vi "Log Data.vi"(0 "Log Data":bool[](array[boolean]), 1 "Log AKLH":bool[](array[boolean]), 2 "Data Log Dirs":path[](array[path]), 3 "AKLH Today Dirs":path[](array[path]), 4 "Record Time (sec)":dbl, 5 "Target Speed":u16, 6 "Test Profile":T4[](array[typedef]) {"Pump Cmds"."Pump 6\nCmd" min=0 format="%#.1f"; "Pump Cmds"."Pump 5\nCmd" min=0 format="%#.1f"; "Pump Cmds"."Pump 4\nCmd" min=0 format="%#.1f"; "Pump Cmds"."Pump 3\nCmd" min=0 format="%#.1f"; "Pump Cmds"."Pump 2\nCmd" min=0 format="%#.1f"; "Pump Cmds"."Pump 1\nCmd" min=0 format="%#.1f"; "Temp\nCmd" min=-60 max=100; "Pressure\nCmd" max=20; "PS\nCmd" min=0 max=20 format="%#.2f"; "Time (s)" min=0.0 step=0.01 format="%#.2g"}, 7 "Current Step":i32=2, 8 "Pump Data":T3={"Voltages"=[0.015201568603515625, 0.00335693359375, 0.003021240234375, 0.12260055541992188, 0.06085968017578125, 0.052234649658203125], "PumpCurrent"=[0.015201568603515625, 0.00335693359375, 0.003021240234375, 0.12260055541992188, 0.06085968017578125, 0.052234649658203125], "Speed"=[0.0, 0.0, 0.0, 0.0, 0.0, 0.0], "ControllerCurrent"=[0.015201568603515625, 0.00335693359375, 0.003021240234375, 0.12260055541992188, 0.06085968017578125, 0.052234649658203125], "Pressure"=[0.015201568603515625, 0.00335693359375, 0.003021240234375, 0.12260055541992188, 0.06085968017578125, 0.052234649658203125], "Flow"=[0.0, 0.0, 0.0, 0.125, 0.0625, 0.0625], "Elapsed Time (Display)"=[7.1, 7.1, 7.1, 458133.45, 458138.85000000003, 458126.75], "Avg Pressure"=0.0, "Avg Speed"=0.0, "Elapsed Time"=[4074.9003000000002, 4074.9003000000002, 4074.9003000000002, 4074.9003000000002, 4074.9003000000002, 4074.9003000000002], "Diagnostic"=[0.0, 0.0, 0.0, 0.0, 0.0, 0.0]} {"Diagnostic" format="%#.0f"; "Elapsed Time" format="%<%H:%M:%S>t"; "Elapsed Time (Display)" format="%<%H:%M:%S>t"; "Speed" format="%#_4f"; "ControllerCurrent" format="%#.1g"; "Pressure" format="%#.0f"; "Flow" format="%#.0f"; "PumpCurrent" format="%#.1g"; "Voltages" format="%#.0f"}, 9 "Tank CMDs":T1, 10 "Tank Data":T2 {"PS Actual (V):" format="%.2f"; "Temp1" format="%#_2g"; "Temp2" format="%#_2g"}, 11 "AKLH Filename":string, 13 "3 Pump Tank":bool) -> ()   [LabVIEW 2019]
uses:
  Type Defs/Test Step.ctl
  Type Defs/Pump Cmds.ctl
  Controls/Pump Data.ctl
  Controls/Tank Data.ctl
  Controls/Tank CMDs.ctl
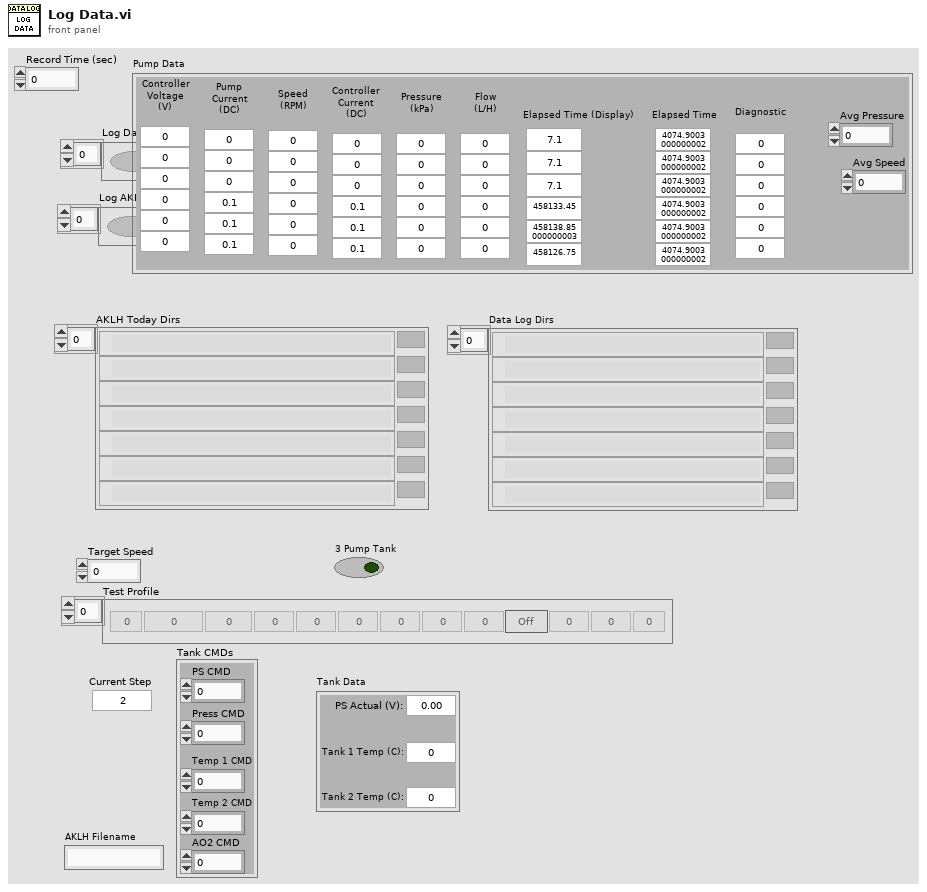
[diagram p1: front panel]
types:
  T1 = typedef "Tank CMDs.ctl" = cluster{"PS CMD":dbl, "Press CMD":dbl, "Temp 1 CMD":dbl, "Temp 2 CMD":dbl, "AO2 CMD":dbl}
  T2 = typedef "Tank Data.ctl" = cluster{"PS Actual (V):":dbl, "Temp1":dbl, "Temp2":dbl}
  T3 = typedef "Pump Data.ctl" = cluster{"Voltages":dbl[], "PumpCurrent":dbl[], "Speed":dbl[], "ControllerCurrent":dbl[], "Pressure":dbl[], "Flow":dbl[], "Elapsed Time (Display)":dbl[], "Avg Pressure":dbl, "Avg Speed":dbl, "Elapsed Time":dbl[], "Diagnostic":dbl[]}
  T4 = typedef "Test Step.ctl" = cluster{"Step":u8, "Time (s)":dbl, "Target\nSpeed":u16, "Pump Cmds":T5, "Relays":bool, "PS\nCmd":sgl, "Pressure\nCmd":u16, "Temp\nCmd":i16}
  T5 = typedef "Pump Cmds.ctl" = cluster{"Pump 1\nCmd":sgl, "Pump 2\nCmd":sgl, "Pump 3\nCmd":sgl, "Pump 4\nCmd":sgl, "Pump 5\nCmd":sgl, "Pump 6\nCmd":sgl}
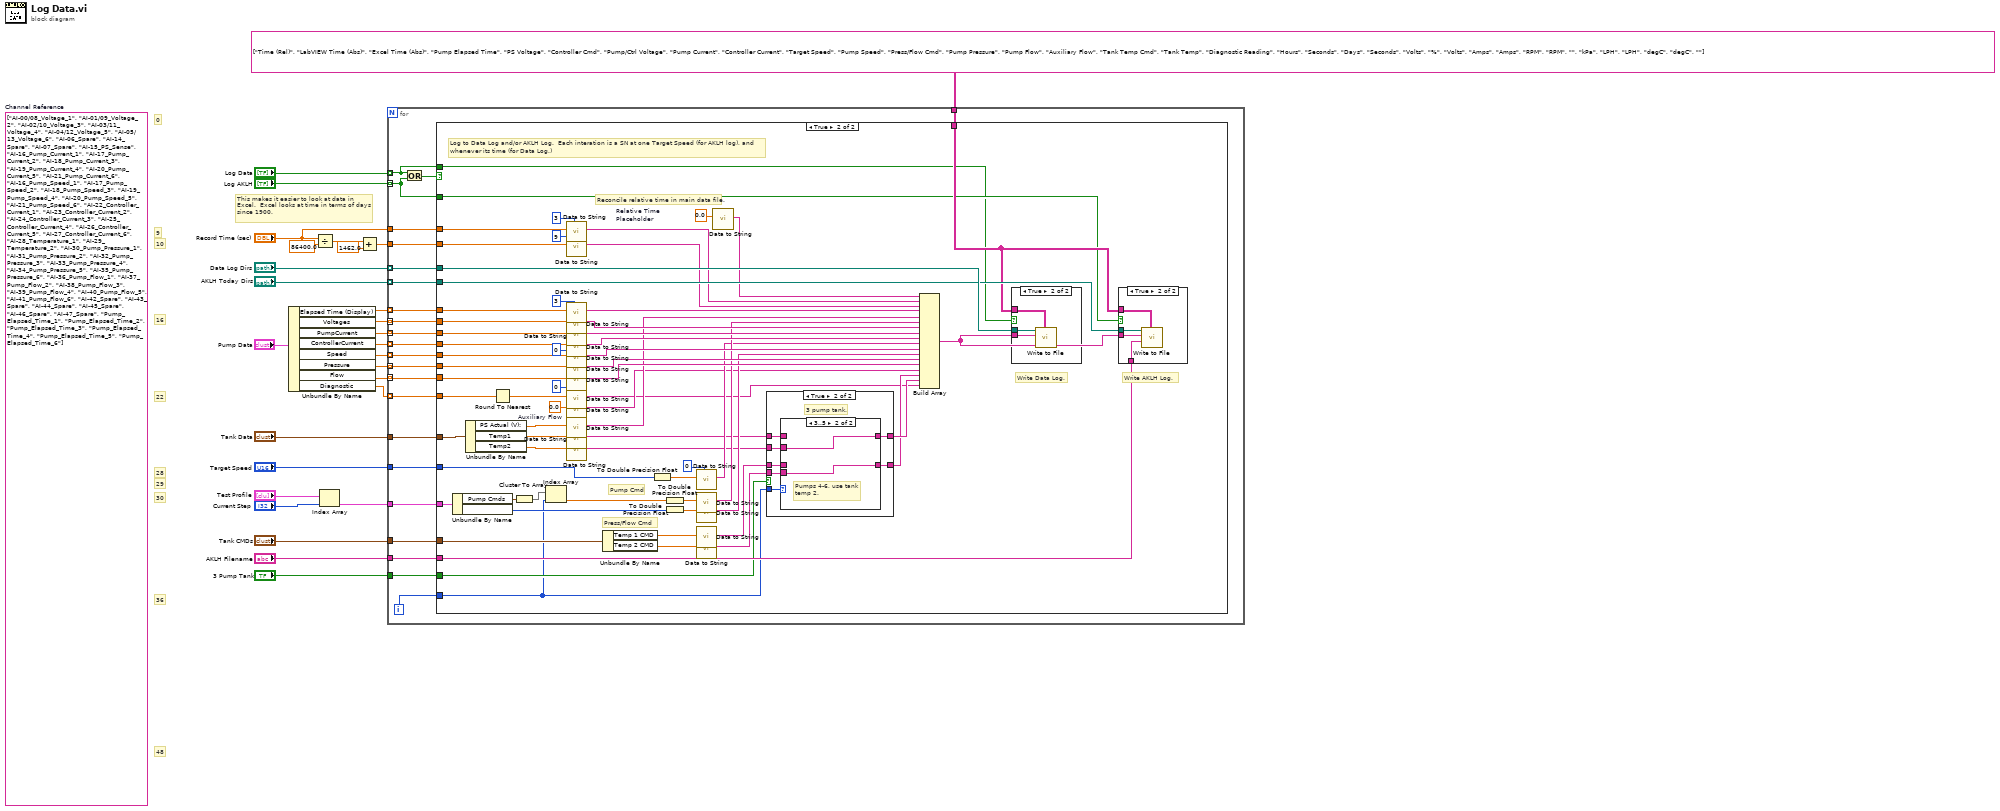
[diagram p0: block diagram]
diagram:
  (unwired) string[] ["AI-00/08_Voltage_1", "AI-01/09_Voltage_2", "AI-02/10_Voltage_3", "AI-03/11_Voltage_4", "AI-04/12_Voltage_5", "AI-05/13_Voltage_6", "AI-06_Spare", "AI-14_Spare", "AI-07_Spare", "AI-15_PS_Sense", "AI-16_Pump_Current_1", "AI-17_Pump_Current_2", "AI-18_Pump_Current_3", "AI-19_Pump_Current_4", "AI-20_Pump_Current_5", "AI-21_Pump_Current_6", "AI-16_Pump_Speed_1", "AI-17_Pump_Speed_2", "AI-18_Pump_Speed_3", "AI-19_Pump_Speed_4", "AI-20_Pump_Speed_5", "AI-21_Pump_Speed_6", "AI-22_Controller_Current_1", "AI-23_Controller_Current_2", "AI-24_Controller_Current_3", "AI-25_Controller_Current_4", "AI-26_Controller_Current_5", "AI-27_Controller_Current_6", "AI-28_Temperature_1", "AI-29_Temperature_2", "AI-30_Pump_Pressure_1", "AI-31_Pump_Pressure_2", "AI-32_Pump_Pressure_3", "AI-33_Pump_Pressure_4", "AI-34_Pump_Pressure_5", "AI-35_Pump_Pressure_6", "AI-36_Pump_Flow_1", "AI-37_Pump_Flow_2", "AI-38_Pump_Flow_3", "AI-39_Pump_Flow_4", "AI-40_Pump_Flow_5", "AI-41_Pump_Flow_6", "AI-42_Spare", "AI-43_Spare", "AI-44_Spare", "AI-45_Spare", "AI-46_Spare", "AI-47_Spare", "Pump_Elapsed_Time_1", "Pump_Elapsed_Time_2", "Pump_Elapsed_Time_3", "Pump_Elapsed_Time_4", "Pump_Elapsed_Time_5", "Pump_Elapsed_Time_6"]  # Channel Reference
  # "This makes it easier to look at data in\nExcel.  Excel looks at time in terms of days\nsince 1900."
  # "36"
  # "30"
  # "29"
  # "28"
  # "22"
  # "16"
  # "10"
  # "9"
  # "0"
  # "48"
  n1 = Unbundle By Name("Pump Data") -> ("Elapsed Time (Display)"=w18:dbl[], "Voltages"=w17:dbl[], "PumpCurrent"=w16:dbl[], "ControllerCurrent"=w15:dbl[], "Speed"=w14:dbl[], "Pressure"=w13:dbl[], "Flow"=w12:dbl[], "Diagnostic"=w3:dbl[])
  n2 = Divide(x="Record Time (sec)", y=86400.0) -> (x/y=w8:dbl)
  n3 = Index Array(array="Test Profile", index="Current Step") -> (element=w1:T4)
  n4 = Add(x=w8, y=1462.0) -> (x+y=w5:dbl)
  n5 = for {
    tunnel: "Data Log Dirs" -> [w50] mode=indexing
    tunnel: "AKLH Today Dirs" -> [w49] mode=indexing
    tunnel: "Record Time (sec)" -> [w48]
    tunnel: "AKLH Filename" -> [w46]
    tunnel: "Target Speed" -> [w45]
    tunnel: "Tank CMDs" -> [w44]
    tunnel: string[][] [["Time (Rel)", "LabVIEW Time (Abs)", "Excel Time (Abs)", "Pump Elapsed Time", "PS Voltage", "Controller Cmd", "Pump/Ctrl Voltage", "Pump Current", "Controller Current", "Target Speed", "Pump Speed", "Press/Flow Cmd", "Pump Pressure", "Pump Flow", "Auxiliary Flow", "Tank Temp Cmd", "Tank Temp", "Diagnostic Reading"], ["Hours", "Seconds", "Days", "Seconds", "Volts", "%", "Volts", "Amps", "Amps", "RPM", "RPM", "", "kPa", "LPH", "LPH", "degC", "degC", ""]] ("subarray") -> [w43]
    tunnel: "Log Data" -> [w41] mode=indexing
    tunnel: "Log AKLH" -> [w40] mode=indexing
    tunnel: w18 -> [w38] mode=indexing
    tunnel: w17 -> [w37] mode=indexing
    tunnel: w16 -> [w36] mode=indexing
    tunnel: w15 -> [w35] mode=indexing
    tunnel: w14 -> [w34] mode=indexing
    tunnel: w13 -> [w33] mode=indexing
    tunnel: w12 -> [w32] mode=indexing
    tunnel: "Tank Data" -> [w39]
    tunnel: w5 -> [w31]
    tunnel: "3 Pump Tank" -> [w30]
    tunnel: w3 -> [w29] mode=indexing
    tunnel: w1 -> [w28]
    i -> [w47]
    n6 = Or(x=w41, y=w40) -> (x .or. y?=w42:bool)
    n7 = case shown="True" w42 {
      tunnel: w50 -> [_ w115]
      tunnel: w49 -> [_ w114]
      tunnel: w48 -> [_ w107]
      tunnel: w41 -> [_ w109]
      tunnel: w47 -> [_ w55]
      tunnel: w46 -> [_ w111]
      tunnel: w45 -> [_ w60]
      tunnel: w44 -> [_ w116]
      tunnel: w43 -> [_ w113]
      tunnel: w40 -> [_ w110]
      tunnel: w39 -> [_ w108]
      tunnel: w38 -> [_ w102]
      tunnel: w37 -> [_ w96]
      tunnel: w36 -> [_ w94]
      tunnel: w35 -> [_ w92]
      tunnel: w34 -> [_ w90]
      tunnel: w33 -> [_ w87]
      tunnel: w32 -> [_ w85]
      tunnel: w31 -> [_ w105]
      tunnel: w30 -> [_ w73]
      tunnel: w29 -> [_ w68]
      tunnel: w28 -> [_ w58]
      frame False {
        # "Neither Data Log is ready to log, nor pump in spec."
      }
      frame True {
        w61 = 0.0  # Auxiliary Flow
        w98 = 0.0  # Relative Time Placeholder
        # "Press/Flow Cmd"
        # "Pump Cmd"
        # "Reconcile relative time in main data file."
        # "Write AKLH Log."
        # "Write Data Log."
        # "Log to Data Log and/or AKLH Log.  Each interation is a SN at one Target Speed (for AKLH log), and\nwhenever its time (for Data Log.)"
        n8 = Unbundle By Name(w58) -> ("Pump Cmds"=w56:T5, "Pressure\nCmd"=w57:u16)
        n9 = Unbundle By Name(w108) -> ("PS Actual (V):"=w83:dbl, "Temp1"=w81:dbl, "Temp2"=w80:dbl)
        n10 = Round To Nearest(number=w68) -> (nearest integer value=w63:dbl)
        n11 = Cluster To Array(cluster=w56) -> (array=w51:sgl[])
        n12 = Index Array(array=w51, index=w55) -> (element=w54:sgl)
        n13 = call "Data to String.vi"("Precision (2)"=i16 3, "Data"=w107) -> ("String Data"=w106:string)  [unwired: 9 in]
        n14 = call "Data to String.vi"("Precision (2)"=i16 9, "Data"=w105) -> ("String Data"=w104:string)  [unwired: 9 in]
        n15 = call "Data to String.vi"("Precision (2)"=i16 3, "Data"=w102) -> ("String Data"=w101:string)  [unwired: 9 in]
        n16 = call "Data to String.vi"("Data"=w96) -> ("String Data"=w95:string)  [unwired: 10 in]
        n17 = call "Data to String.vi"("Data"=w94) -> ("String Data"=w93:string)  [unwired: 10 in]
        n18 = call "Data to String.vi"("Data"=w92) -> ("String Data"=w91:string)  [unwired: 10 in]
        n19 = call "Data to String.vi"("Precision (2)"=i16 0, "Data"=w90) -> ("String Data"=w89:string)  [unwired: 9 in]
        n20 = call "Data to String.vi"("Data"=w87) -> ("String Data"=w86:string)  [unwired: 10 in]
        n21 = call "Data to String.vi"("Data"=w85) -> ("String Data"=w84:string)  [unwired: 10 in]
        n22 = call "Data to String.vi"("Precision (2)"=i16 0, "Data"=w63) -> ("String Data"=w64:string)  [unwired: 9 in]
        n23 = call "Data to String.vi"("Data"=w61) -> ("String Data"=w65:string)  [unwired: 10 in]
        n24 = call "Data to String.vi"("Data"=w83) -> ("String Data"=w82:string)  [unwired: 10 in]
        n25 = call "Data to String.vi"("Data"=w81) -> ("String Data"=w71:string)  [unwired: 10 in]
        n26 = call "Data to String.vi"("Data"=w80) -> ("String Data"=w70:string)  [unwired: 10 in]
        n27 = Unbundle By Name(w116) -> ("Temp 1 CMD"=w77:dbl, "Temp 2 CMD"=w76:dbl)
        n28 = To Double Precision Float(number=w60) -> (double precision float=w59:dbl)
        n29 = To Double Precision Float(number=w54) -> (double precision float=w53:dbl)
        n30 = To Double Precision Float(number=w57) -> (double precision float=w52:dbl)
        n31 = call "Data to String.vi"("Precision (2)"=i16 0, "Data"=w59) -> ("String Data"=w74:string)  [unwired: 9 in]
        n32 = call "Data to String.vi"("Data"=w53) -> ("String Data"=w79:string)  [unwired: 10 in]
        n33 = call "Data to String.vi"("Data"=w52) -> ("String Data"=w78:string)  [unwired: 10 in]
        n34 = call "Data to String.vi"("Data"=w77) -> ("String Data"=w72:string)  [unwired: 10 in]
        n35 = call "Data to String.vi"("Data"=w76) -> ("String Data"=w69:string)  [unwired: 10 in]
        n36 = call "Data to String.vi"("Data"=w98) -> ("String Data"=w97:string)  [unwired: 10 in]
        n37 = case shown="True" w73 {
          tunnel: w72 -> [w118 w122]
          tunnel: [w118 w121] -> w66
          tunnel: [w117 w123] -> w67
          tunnel: w71 -> [w117 w124]
          tunnel: w55 -> [_ w125]
          tunnel: w70 -> [_ w120]
          tunnel: w69 -> [_ w119]
          frame False {
            # "Only one tank, so use\ntank temp 1."
            # "6 pump tank."
          }
          frame True {
            # "3 pump tank."
            n38 = case shown="3..5" w125 {
              tunnel: [w127 w129] -> w123
              tunnel: w124 -> [w127 _]
              tunnel: [w126 w128] -> w121
              tunnel: w122 -> [w126 _]
              tunnel: w120 -> [_ w129]
              tunnel: w119 -> [_ w128]
              frame 0..2, Default {
                # "Pumps 1-3, use tank\ntemp 1."
              }
              frame 3..5 {
                # "Pumps 4-6, use tank\ntemp 2."
              }
            }
          }
        }
        n39 = Build Array(w97, w106, w104, w101, w82, w79, w95, w93, w91, w74, w89, w78, w86, w84, w65, w66, w67, w64) -> (w112:string[])
        n40 = case shown="True" w109 {
          tunnel: w115 -> [_ w136]
          tunnel: w113 -> [_ w135]
          tunnel: w112 -> [_ w134]
          frame False {
          }
          frame True {
            n41 = call "Write to File.vi"("Column Header"=w135, "Data"=w134, "Path"=w136) -> ()  [unwired: 9 in]
          }
        }
        n42 = case shown="True" w110 {
          tunnel: w114 -> [_ w133]
          tunnel: w113 -> [_ w132]
          tunnel: w112 -> [_ w131]
          tunnel: w111 -> [_ w130]
          frame False {
          }
          frame True {
            n43 = call "Write to File.vi"("Column Header"=w132, "Filename"=w130, "Data"=w131, "Path"=w133) -> ()  [unwired: 8 in]
          }
        }
      }
    }
  }
